vi "exercise4.vi"() -> ()   [LabVIEW 2025]
panel:
  in  "SI":bool
  in  "LA":bool
  in  "SOL":bool
  in  "FA":bool
  in  "MI":bool
  in  "RE":bool
  in  "DO":bool
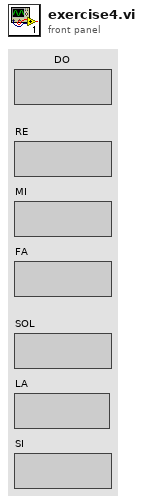
[diagram p1: front panel]
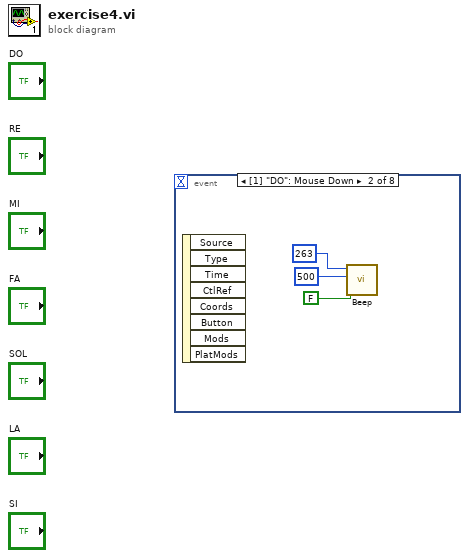
[diagram p0: block diagram]
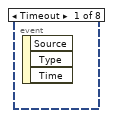
[diagram p2: hidden frame]
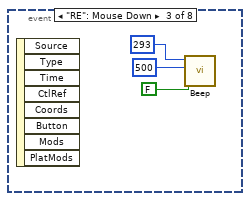
[diagram p3: hidden frame]
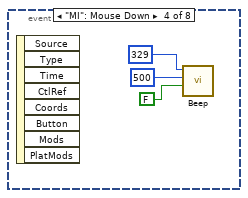
[diagram p4: hidden frame]
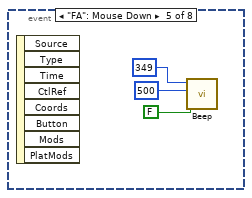
[diagram p5: hidden frame]
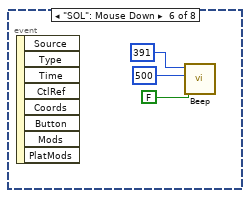
[diagram p6: hidden frame]
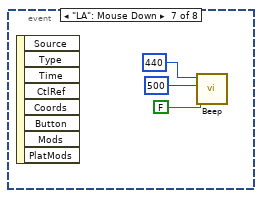
[diagram p7: hidden frame]
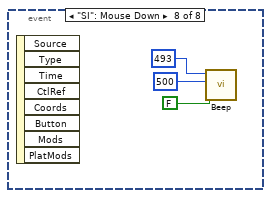
[diagram p8: hidden frame]
diagram:
  n1 = event shown="[1] \"DO\": Mouse Down" {
    selector: _ -> [_ _ _ _ _ _ _ _]
    dyn-events: _ -> [_ _ _ _ _ _ _ _]
    timeout: _ -> [_ _ _ _ _ _ _ _]
    event Timeout {
      n2 = event-data() -> ()  [unwired: 1 in, 3 out]
    }
    event "DO": Mouse Down {
      n3 = event-data() -> ()  [unwired: 1 in, 8 out]
      n4 = call <vilib>:"Beep.vi"("use system alert? (T)"=FALSE, "duration (msec)"=u32 500, "frequency (Hz)"=u32 263) -> ()  [unwired: 9 in]
    }
    event "RE": Mouse Down {
      n5 = event-data() -> ()  [unwired: 1 in, 8 out]
      n6 = call <vilib>:"Beep.vi"("use system alert? (T)"=FALSE, "duration (msec)"=u32 500, "frequency (Hz)"=u32 293) -> ()  [unwired: 9 in]
    }
    event "MI": Mouse Down {
      n7 = event-data() -> ()  [unwired: 1 in, 8 out]
      n8 = call <vilib>:"Beep.vi"("use system alert? (T)"=FALSE, "duration (msec)"=u32 500, "frequency (Hz)"=u32 329) -> ()  [unwired: 9 in]
    }
    event "FA": Mouse Down {
      n9 = event-data() -> ()  [unwired: 1 in, 8 out]
      n10 = call <vilib>:"Beep.vi"("use system alert? (T)"=FALSE, "duration (msec)"=u32 500, "frequency (Hz)"=u32 349) -> ()  [unwired: 9 in]
    }
    event "SOL": Mouse Down {
      n11 = event-data() -> ()  [unwired: 1 in, 8 out]
      n12 = call <vilib>:"Beep.vi"("use system alert? (T)"=FALSE, "duration (msec)"=u32 500, "frequency (Hz)"=u32 391) -> ()  [unwired: 9 in]
    }
    event "LA": Mouse Down {
      n13 = event-data() -> ()  [unwired: 1 in, 8 out]
      n14 = call <vilib>:"Beep.vi"("use system alert? (T)"=FALSE, "duration (msec)"=u32 500, "frequency (Hz)"=u32 440) -> ()  [unwired: 9 in]
    }
    event "SI": Mouse Down {
      n15 = event-data() -> ()  [unwired: 1 in, 8 out]
      n16 = call <vilib>:"Beep.vi"("use system alert? (T)"=FALSE, "duration (msec)"=u32 500, "frequency (Hz)"=u32 493) -> ()  [unwired: 9 in]
    }
  }
